vi "TIC_write.vi"(2 "error in (no error)":errorcluster, 3 "write buffer":string, 4 "TIC 500":refnum<visa-resource-name>="COM6") -> (0 "error out":errorcluster, 1 "VISA resource name out":refnum<visa-resource-name>="COM6")   [LabVIEW 2011]
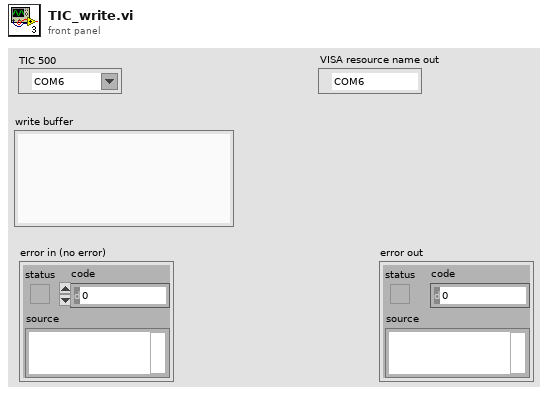
[diagram p1: front panel]
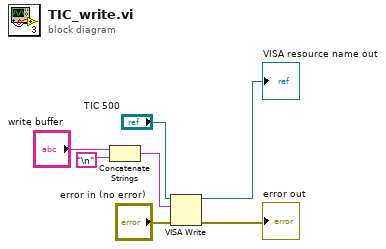
[diagram p0: block diagram]
diagram:
  n1 = Concatenate Strings("write buffer", "\n") -> (w3:string)
  n2 = VISA Write(VISA resource name="TIC 500", write buffer=w3, error in (no error)="error in (no error)") -> (VISA resource name out=→"VISA resource name out":refnum<visa-resource-name>, error out=→"error out":errorcluster)  [unwired: 1 out]
